vi "Normalize Coordinates.vi"(6 "Score":dbl, 9 "Distance":dbl, 10 "Bounding box":T3, 11 "Image in":T1) -> (1 "Results":T2 {"Score" format="%#_3g"; "Pixels"."Rectangle"."Numeric 5" format="%#_3g"; "Pixels"."Rectangle"."Numeric 3" format="%#_3g"; "Pixels"."Rectangle"."Numeric 2" format="%#_3g"; "Pixels"."Rectangle"."Numeric" format="%#_3g"; "Normalized"."Rectangle"."Numeric 5" format="%#_2g"; "Normalized"."Rectangle"."Numeric 3" format="%#_2g"; "Normalized"."Rectangle"."Numeric 2" format="%#_2g"; "Normalized"."Rectangle"."Numeric" format="%#_2g"; "Normalized"."Center"."?" format="%#_3g"; "Normalized"."Center"."?" format="%#_3g"; "Distance (ft)" format="%#_3g"}, 3 "Image out":T1)   [LabVIEW 2018]
doc: "Normalize the rectangle and center so that they range from -1 to 1, left to right and bottom to top. This helps with producing joystick coordinates for driving the robot and makes the code better at handling resolution changes of the camera."
uses:
  <vilib>/vision/Image Controls.llb/IMAQ Image.ctl
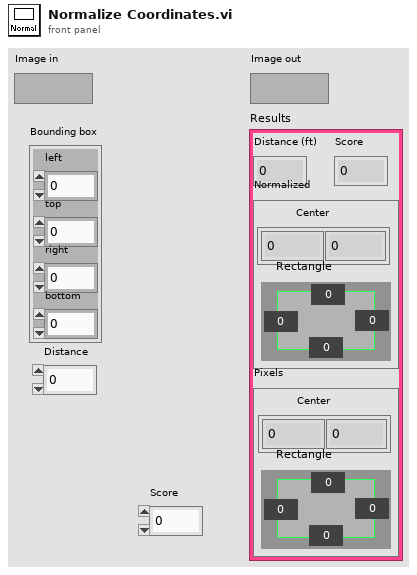
[diagram p1: front panel]
types:
  T1 = typedef "IMAQ Image.ctl" = refnum<image>
  T2 = cluster{"Distance (ft)":dbl, "Score":dbl, "Normalized":cluster{"Center":cluster{dbl, dbl}, "Rectangle":cluster{"Numeric":dbl, "Numeric 2":dbl, "Numeric 3":dbl, "Numeric 5":dbl}}, "Pixels":cluster{"Center":cluster{dbl, dbl}, "Rectangle":cluster{"Numeric":dbl, "Numeric 2":dbl, "Numeric 3":dbl, "Numeric 5":dbl}}}
  T3 = cluster{"left":dbl, "top":dbl, "right":dbl, "bottom":dbl}
  T4 = cluster{"X Resolution":i32, i32, "X Resolution":i32, i32}
  T5 = cluster{cluster{dbl, dbl}, "Bounding box":cluster{"left":dbl, "top":dbl, "right":dbl, "bottom":dbl}}
  T6 = cluster{cluster{dbl, dbl}, cluster{dbl, dbl, dbl, dbl}}
  T7 = cluster{"Distance":dbl, "Score":dbl, cluster{cluster{dbl, dbl}, cluster{dbl, dbl, dbl, dbl}}, cluster{cluster{dbl, dbl}, "Bounding box":cluster{"left":dbl, "top":dbl, "right":dbl, "bottom":dbl}}}
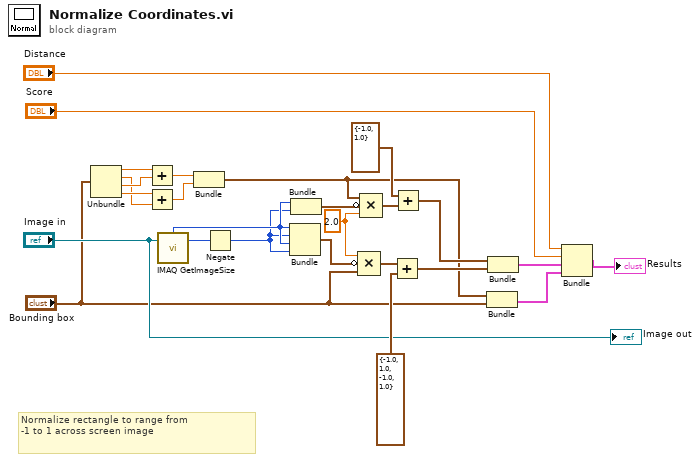
[diagram p0: block diagram]
diagram:
  w14 = 2.0
  # "Normalize rectangle to range from\n-1 to 1 across screen image"
  n1 = Unbundle("Bounding box") -> ("left"=w7:dbl, "top"=w4:dbl, "right"=w6:dbl, "bottom"=w5:dbl)
  n2 = Add(x=w7, y=w6) -> (x+y=w3:dbl)
  n3 = Add(x=w5, y=w4) -> (x+y=w2:dbl)
  n4 = call "IMAQ GetImageSize"("Image"="Image in") -> ("Y Resolution"=w26:i32, "X Resolution"=w17:i32)  [unwired: 3 in, 1 out]
  n5 = Bundle(w3, w2) -> (w1:cluster{dbl, dbl})  [unwired: 1 in]
  n6 = Negate(x=w26) -> (-x=w16:i32)
  n7 = Bundle("X Resolution"=w17, w16, "X Resolution"=w17, w16) -> (w24:T4)  [unwired: 1 in]
  n8 = Bundle("X Resolution"=w17, w16) -> (w15:cluster{"X Resolution":i32, i32})  [unwired: 1 in]
  n9 = Compound Arithmetic op=MULTIPLY(w14, invert w24, "Bounding box") -> (w23:cluster{dbl, dbl, dbl, dbl})
  n10 = Compound Arithmetic op=MULTIPLY(w1, invert w15, w14) -> (w13:cluster{dbl, dbl})
  n11 = Add(x=w23, y=cluster{dbl, dbl, dbl, dbl} {-1.0, 1.0, -1.0, 1.0}) -> (x+y=w22:cluster{dbl, dbl, dbl, dbl})
  n12 = Add(x=cluster{dbl, dbl} {-1.0, 1.0} ("y"), y=w13) -> (x+y=w12:cluster{dbl, dbl})
  n13 = Bundle(w1, "Bounding box"="Bounding box") -> (w18:T5)  [unwired: 1 in]
  n14 = Bundle(w12, w22) -> (w20:T6)  [unwired: 1 in]
  n15 = Bundle("Distance"="Distance", "Score"="Score", w20, w18) -> (→"Results":T7)  [unwired: 1 in]
  "Image out" <- "Image in"
